vi "质控单元MB_api.vi"(6 "Slave ID":u8=1, 7 "STEP":enum16{"open", "read", "write", "close"}(ring)=enum."read", 8 "Error in":errorcluster caption="Error in (no error)", 9 "values":u16[](array[numeric]), 10 "quantity":u16, 11 "starting address":u16 format="%04xH") -> (0 "error out":errorcluster, 1 "MB session out":refnum<class "MB_Master.lvclass">, 3 "Registers":u16[](array[numeric]))   [LabVIEW 2016, in "质控单元.lvlib"]
uses:
  <vilib>/Plasmionique/MB Master/MB_Master/MB_Master.lvclass
  <vilib>/Plasmionique/MB Master/MB_Master_Serial/MB_Master_Serial.lvclass
  D:/Program Files (x86)/National Instruments/LabVIEW 2016/vi.lib/Plasmionique/MB Master/MB_Master/MB_Master.lvclass
  <vilib>/Plasmionique/MB Master/MB_Master_TCP/MB_Master_TCP.lvclass
  <vilib>/Plasmionique/MB Master/MB Master.lvlib
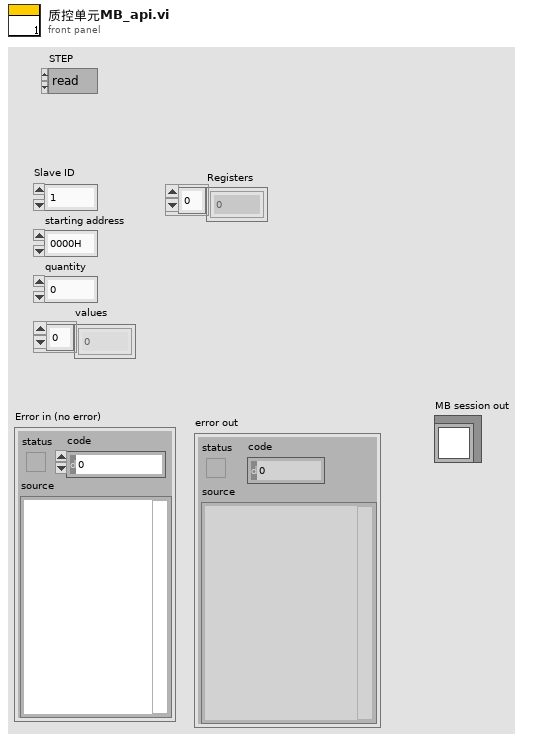
[diagram p1: front panel]
types:
  T1 = cluster{"baud rate (bps)":u32, "stop bits":u16, "parity":u16, "flow control":u16, "timeout":u32, "retries":i32}
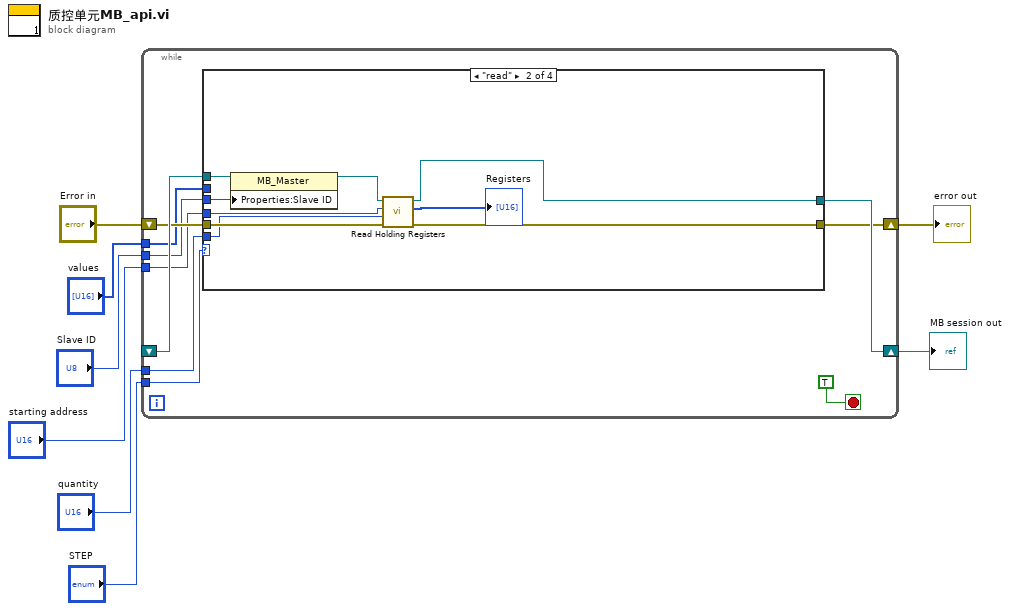
[diagram p0: block diagram]
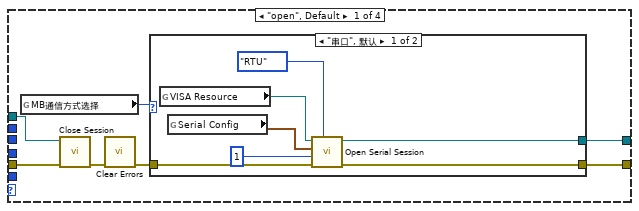
[diagram p2: hidden frame]
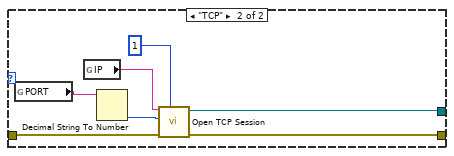
[diagram p3: hidden frame]
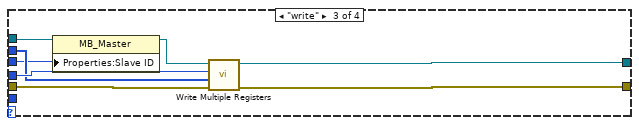
[diagram p4: hidden frame]
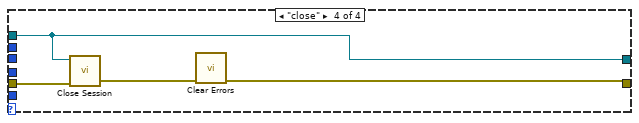
[diagram p5: hidden frame]
diagram:
  n1 = while {
    shift-right: [w12] -> w1
    shift-left: _ -> [w18]
    shift-right: [w11] -> w7
    shift-left: "Error in" -> [w17]
    tunnel: "Slave ID" -> [w16]
    tunnel: "starting address" -> [w15]
    tunnel: "quantity" -> [w14]
    tunnel: "STEP" -> [w13]
    tunnel: "values" -> [w10]
    stop <- TRUE stop-if-true
    n2 = case shown="\"read\"" w13 {
      tunnel: w18 -> [w23 w41 w51 w59]
      tunnel: w17 -> [w22 w48 w56 w60]
      tunnel: [w24 w47 w54 w59] -> w12
      tunnel: [w25 w46 w55 w57] -> w11
      tunnel: w16 -> [_ w44 w50 _]
      tunnel: w15 -> [_ w43 w53 _]
      tunnel: w14 -> [_ w42 _ _]
      tunnel: w10 -> [_ _ w52 _]
      frame "open", Default {
        n3 = global read "断电保存全局.vi" "MB通信方式选择"() -> (w19:enum16{"串口", "TCP"})
        n4 = call-dynamic "Close Session.vi"("error in (no error)"=w22, "MB session in"=w23) -> ("error out"=w21:errorcluster)  [unwired: 9 in]
        n5 = call <vilib>:"Clear Errors.vi"("error in (no error)"=w21) -> ("error out"=w20:errorcluster)  [unwired: 5 in, 1 out]
        n6 = case shown="\"串口\", 默认" w19 {
          tunnel: [w31 w36] -> w25
          tunnel: [w27 w34] -> w24
          tunnel: w20 -> [w28 w35]
          frame "串口", Default {
            n7 = global read "断电保存全局.vi" "VISA Resource"() -> (w30:refnum<visa-resource-name>)
            n8 = global read "断电保存全局.vi" "Serial Config"() -> (w29:T1)
            n9 = call <vilib>:"Open Serial Session.vi"("Mode (RTU)"=enum16{"RTU", "ASCII"}."RTU", "Error in"=w28, "Slave ID"=u8 1, "Serial Config"=w29, "VISA Resource"=w30) -> ("Error out"=w31:errorcluster, "MB_Serial session"=w27:refnum<class "MB_Master_Serial.lvclass">)  [unwired: 5 in]
          }
          frame "TCP" {
            n10 = global read "断电保存全局.vi" "PORT"() -> (w38:string)
            n11 = global read "断电保存全局.vi" "IP"() -> (w37:string)
            n12 = Decimal String To Number(string=w38) -> (number=w39:i32)  [unwired: 2 in, 1 out]
            n13 = call <vilib>:"Open TCP Session.vi"("Slave ID (255)"=u8 1 ("Slave ID"), "error in (no error)"=w35, "Port (502)"=w39, "IP Address"=w37) -> ("error out"=w36:errorcluster, "MB_TCP session"=w34:refnum<class "MB_Master_TCP.lvclass">)  [unwired: 6 in]
          }
        }
      }
      frame "read" {
        n14 = property class="MB_Master"(reference=w41, "Properties:Slave ID"=w44) -> (reference out=w40:refnum<class "MB_Master.lvclass">)  [unwired: 1 in, 1 out]
        n15 = call <vilib>:"Read Holding Registers.vi"("error in (no error)"=w48, "quantity"=w42, "starting address"=w43, "MB session in"=w40) -> ("error out"=w46:errorcluster, "Registers"=→"Registers":u16[], "MB session out"=w47:refnum<class "MB_Master.lvclass">)  [unwired: 5 in]
      }
      frame "write" {
        n16 = property class="MB_Master"(reference=w51, "Properties:Slave ID"=w50) -> (reference out=w49:refnum<class "MB_Master.lvclass">)  [unwired: 1 in, 1 out]
        n17 = call <vilib>:"Write Multiple Registers.vi"("error in (no error)"=w56, "values"=w52, "starting address"=w53, "MB session in"=w49) -> ("error out"=w55:errorcluster, "MB session out"=w54:refnum<class "MB_Master.lvclass">)  [unwired: 6 in]
      }
      frame "close" {
        n18 = call-dynamic "Close Session.vi"("error in (no error)"=w60, "MB session in"=w59) -> ("error out"=w58:errorcluster)  [unwired: 9 in]
        n19 = call <vilib>:"Clear Errors.vi"("error in (no error)"=w58) -> ("error out"=w57:errorcluster)  [unwired: 5 in, 1 out]
      }
    }
  }
  "error out" <- w7
  "MB session out" <- w1
